vi "users format permissions from POST.vi"(4 "Edit Admin? (f)":bool, 6 "THE Admin? (f)":bool, 8 "error in (no error)":errorcluster, 9 "Permissions to Edit (F)":T1, 10 "Current User Permissions (F)":T1, 11 "POST (empty)":T2) -> (0 "error out":errorcluster, 3 "User Record":T1)   [LabVIEW 2011]
uses:
  server/database/Users/User Record.ctl
  Addons/internet/utils/keyedarr.llb/Keyed Array.ctl
  Addons/internet/utils/strutil.llb/Case Matching.ctl
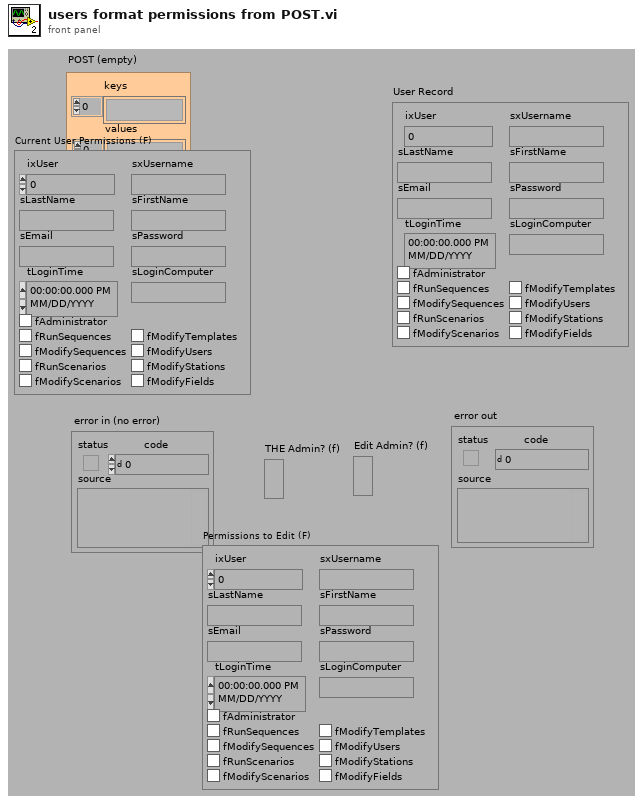
[diagram p1: front panel]
types:
  T1 = typedef "User Record.ctl" = cluster{"ixUser":i32, "sxUsername":string, "sLastName":string, "sFirstName":string, "sEmail":string, "sPassword":string, "tLoginTime":timestamp, "sLoginComputer":string, "fAdministrator":bool, "fRunSequences":bool, "fModifySequences":bool, "fRunScenarios":bool, "fModifyScenarios":bool, "fModifyTemplates":bool, "fModifyUsers":bool, "fModifyStations":bool, "fModifyFields":bool}
  T2 = typedef "Keyed Array.ctl" = cluster{"keys":string[], "values":string[]}
  T3 = typedef "Case Matching.ctl" = enum16{"a != A", "a == A", "system"}
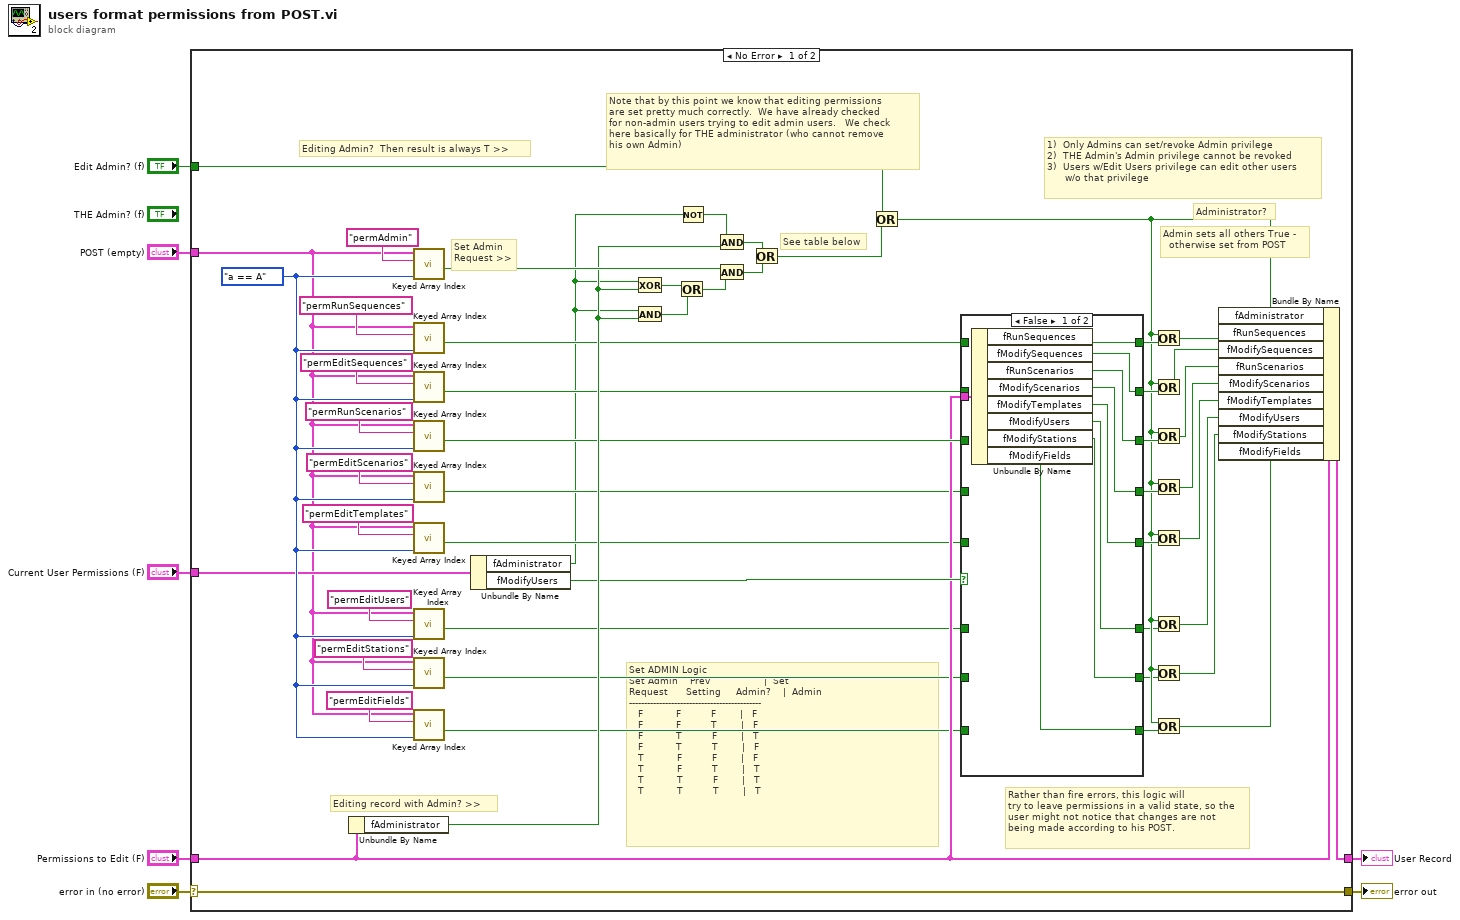
[diagram p0: block diagram]
diagram:
  n1 = case shown="No Error" "error in (no error)" {
    selector: "error in (no error)" -> [w51 w77]
    tunnel: [w52 w78] -> w7
    tunnel: "Permissions to Edit (F)" -> [w33 w78]
    tunnel: [w51 w77] -> w4
    tunnel: "Edit Admin? (f)" -> [w17 _]
    tunnel: "Current User Permissions (F)" -> [w16 _]
    tunnel: "POST (empty)" -> [w15 _]
    frame No Error {
      w30 = Case_Matching."a == A" ("case matching (sensitive)")
      # "Set ADMIN Logic\nSet Admin    Prev                  |  Set\nRequest      Setting     Admin?    |  Admin\n--------------------------------------------\n   F           F          F        |   F\n   F           F          T        |   F\n   F           T          F        |   T\n   F           T          T        |   F\n   T           F          F        |   F\n   T           F          T        |   T\n   T           T          F        |   T\n   T           T          T        |   T"
      # "See table below"
      # "Editing record with Admin? >>"
      # "Set Admin\nRequest >>"
      # "Editing Admin?  Then result is always T >>"
      # "1)  Only Admins can set/revoke Admin privilege\n2)  THE Admin's Admin privilege cannot be revoked\n3)  Users w/Edit Users privilege can edit other users\n      w/o that privilege"
      # "Admin sets all others True -\n  otherwise set from POST"
      # "Note that by this point we know that editing permissions\nare set pretty much correctly.  We have already checked\nfor non-admin users trying to edit admin users.   We check\nhere basically for THE administrator (who cannot remove\nhis own Admin)"
      # "Rather than fire errors, this logic will\ntry to leave permissions in a valid state, so the\nuser might not notice that changes are not\nbeing made according to his POST."
      # "Administrator?"
      n2 = Unbundle By Name(w33) -> ("fAdministrator"=w42:bool)
      n3 = call "Keyed Array Index.vi"("case matching (sensitive)"=w30, "key"="permAdmin", "array in"=w15) -> ("valid key"=w49:bool)  [unwired: 1 in, 3 out]
      n4 = call "Keyed Array Index.vi"("case matching (sensitive)"=w30, "key"="permRunSequences", "array in"=w15) -> ("valid key"=w37:bool)  [unwired: 1 in, 3 out]
      n5 = call "Keyed Array Index.vi"("case matching (sensitive)"=w30, "key"="permEditSequences", "array in"=w15) -> ("valid key"=w38:bool)  [unwired: 1 in, 3 out]
      n6 = call "Keyed Array Index.vi"("case matching (sensitive)"=w30, "key"="permRunScenarios", "array in"=w15) -> ("valid key"=w39:bool)  [unwired: 1 in, 3 out]
      n7 = call "Keyed Array Index.vi"("case matching (sensitive)"=w30, "key"="permEditScenarios", "array in"=w15) -> ("valid key"=w29:bool)  [unwired: 1 in, 3 out]
      n8 = call "Keyed Array Index.vi"("case matching (sensitive)"=w30, "key"="permEditTemplates", "array in"=w15) -> ("valid key"=w28:bool)  [unwired: 1 in, 3 out]
      n9 = call "Keyed Array Index.vi"("case matching (sensitive)"=w30, "key"="permEditUsers", "array in"=w15) -> ("valid key"=w13:bool)  [unwired: 1 in, 3 out]
      n10 = call "Keyed Array Index.vi"("case matching (sensitive)"=w30, "key"="permEditStations", "array in"=w15) -> ("valid key"=w12:bool)  [unwired: 1 in, 3 out]
      n11 = call "Keyed Array Index.vi"("case matching (sensitive)"=w30, "key"="permEditFields", "array in"=w15) -> ("valid key"=w11:bool)  [unwired: 1 in, 3 out]
      n12 = Unbundle By Name(w16) -> ("fAdministrator"=w14:bool, "fModifyUsers"=w40:bool)
      n13 = Exclusive Or(1:w42, 2:w14) -> (0:w48:bool)
      n14 = And(x=w14, y=w42) -> (x .and. y?=w47:bool)
      n15 = Or(x=w48, y=w47) -> (x .or. y?=w46:bool)
      n16 = Not(x=w14) -> (.not. x?=w43:bool)
      n17 = And(x=w43, y=w42) -> (x .and. y?=w44:bool)
      n18 = And(x=w49, y=w46) -> (x .and. y?=w45:bool)
      n19 = Or(x=w44, y=w45) -> (x .or. y?=w41:bool)
      n20 = Or(x=w17, y=w41) -> (x .or. y?=w24:bool)
      n21 = case shown="False" w40 {
        tunnel: w39 -> [_ w74]
        tunnel: w38 -> [_ w75]
        tunnel: w37 -> [_ w76]
        tunnel: [w67 w76] -> w36
        tunnel: [w66 w75] -> w35
        tunnel: [w65 w74] -> w34
        tunnel: w33 -> [w68 _]
        tunnel: w29 -> [_ w72]
        tunnel: w28 -> [_ w73]
        tunnel: [w64 w73] -> w26
        tunnel: [w63 w72] -> w25
        tunnel: w13 -> [_ w69]
        tunnel: w12 -> [_ w70]
        tunnel: w11 -> [_ w71]
        tunnel: [w60 w71] -> w10
        tunnel: [w61 w70] -> w9
        tunnel: [w62 w69] -> w8
        frame False {
          n22 = Unbundle By Name(w68) -> ("fRunSequences"=w67:bool, "fModifySequences"=w66:bool, "fRunScenarios"=w65:bool, "fModifyScenarios"=w63:bool, "fModifyTemplates"=w64:bool, "fModifyUsers"=w62:bool, "fModifyStations"=w61:bool, "fModifyFields"=w60:bool)
        }
        frame True {
        }
      }
      n23 = Or(x=w24, y=w36) -> (x .or. y?=w50:bool)
      n24 = Or(x=w24, y=w35) -> (x .or. y?=w18:bool)
      n25 = Or(x=w24, y=w34) -> (x .or. y?=w27:bool)
      n26 = Or(x=w24, y=w25) -> (x .or. y?=w23:bool)
      n27 = Or(x=w24, y=w26) -> (x .or. y?=w22:bool)
      n28 = Or(x=w24, y=w8) -> (x .or. y?=w20:bool)
      n29 = Or(x=w24, y=w9) -> (x .or. y?=w19:bool)
      n30 = Or(x=w24, y=w10) -> (x .or. y?=w21:bool)
      n31 = Bundle By Name(cluster=w33, "fAdministrator"=w24, "fRunSequences"=w50, "fModifySequences"=w18, "fRunScenarios"=w27, "fModifyScenarios"=w23, "fModifyTemplates"=w22, "fModifyUsers"=w20, "fModifyStations"=w19, "fModifyFields"=w21) -> (w52:T1)
    }
    frame Error {
    }
  }
  "User Record" <- w7
  "error out" <- w4
